vi "CallTransformation.vi"(8 "error in (no error)":errorcluster, 11 "TCP Network Connection in":refnum<k5>) -> (0 "error out":errorcluster, 2 "CallTrafoCluster":T1, 3 "TCP Network Connection out":refnum<k5>, 5 "Respond":string[](array[string]), 7 "Command":string)   [LabVIEW 2017]
uses:
  AT901 API/Structures/Struct CallTrafo.ctl
  AT901 API/TypeDefinitions/ES_DataType.ctl
  AT901 API/TypeDefinitions/ES_Command.ctl
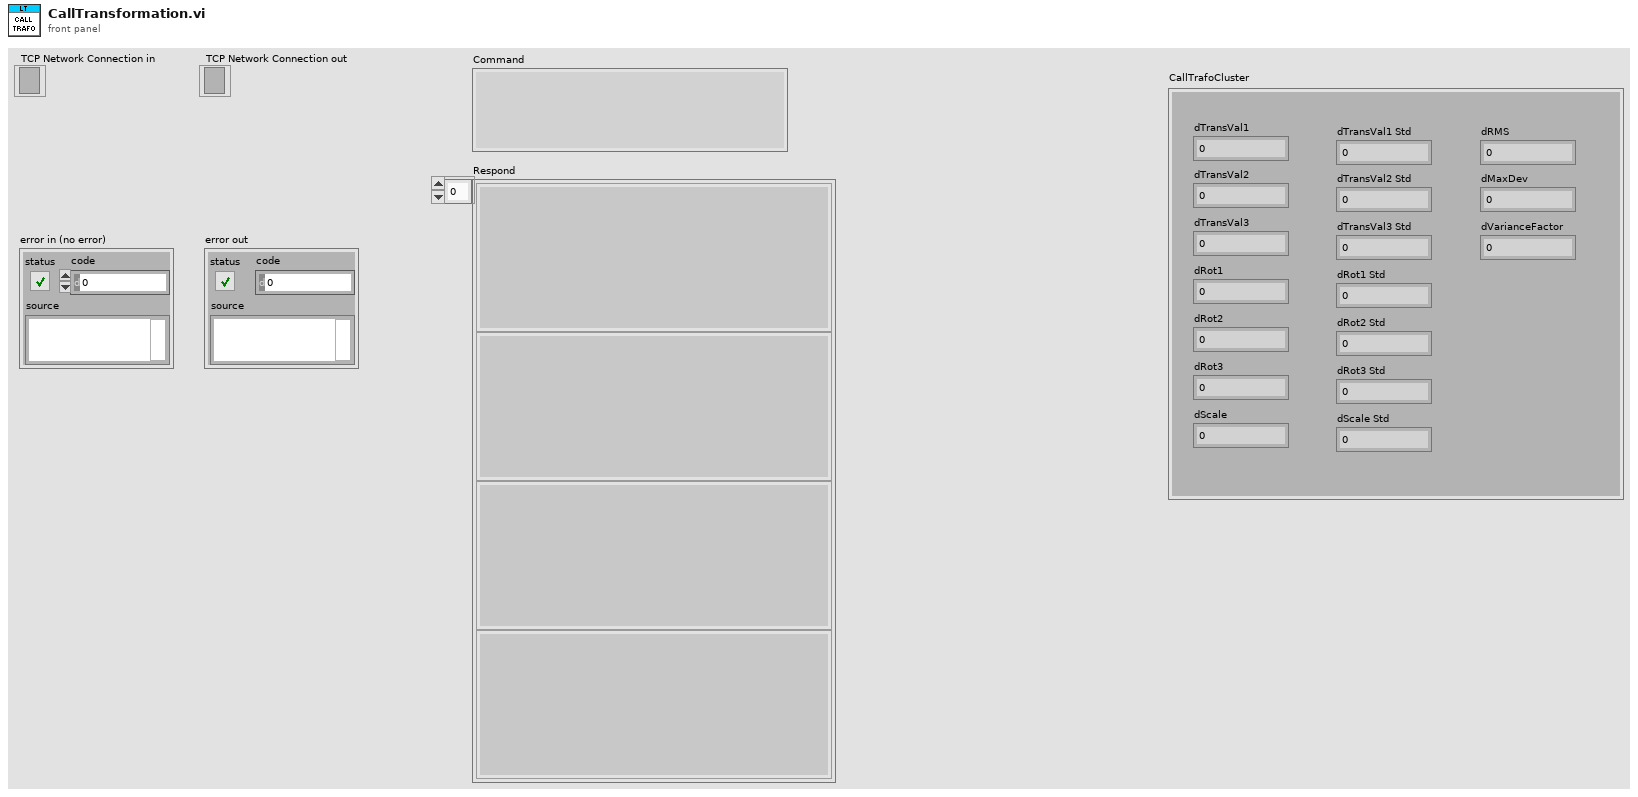
[diagram p1: front panel]
types:
  T1 = typedef "Struct CallTrafo.ctl" = cluster{"dTransVal1":dbl, "dTransVal2":dbl, "dTransVal3":dbl, "dRot1":dbl, "dRot2":dbl, "dRot3":dbl, "dScale":dbl, "dTransVal1 Std":dbl, "dTransVal2 Std":dbl, "dTransVal3 Std":dbl, "dRot1 Std":dbl, "dRot2 Std":dbl, "dRot3 Std":dbl, "dScale Std":dbl, "dRMS":dbl, "dMaxDev":dbl, "dVarianceFactor":dbl}
  T2 = typedef "ES_Command.ctl" = enum32{"ES_C_ExitApplication", "ES_C_GetSystemStatus", "ES_C_GetTrackerStatus", "ES_C_SetTemperatureRange", "ES_C_GetTemperatureRange", "ES_C_SetUnits", "ES_C_GetUnits", "ES_C_Intialize", "ES_C_ReleaseMotors", "ES_C_ActivateCameraView", "ES_C_Park", "ES_C_SwitchLaser", "ES_C_SetStationOriantationParams", "ES_C_GetStationOrientationParams", "ES_C_SetTransformationParams", "ES_C_GetTransformationParams", "ES_C_SetBoxRegionParams", "ES_C_GetBoxRegionParams", "ES_C_SetSphereRegionParams", "ES_C_GetSphereRegionParams", "ES_C_SetEnvironmentParams", "ES_C_GetEnvironmentParams", "ES_C_SetRefractionParams", "ES_C_GetRefractionParams", "ES_C_SetMeasurementMode", "ES_C_GetMeasurementMode", "ES_C_SetCoordinateSystemType", "ES_C_GetCoordinateSystemType", "ES_C_SetStationaryModeParams", "ES_C_GetStationaryModeParams", "ES_C_SetContinuousTimeModeParams", "ES_C_GetContinuousTimeModeParams", "ES_C_SetContinuousDistanceModeParams", "ES_C_GetContinuousDistanceModeParams", "ES_C_SetSphereCenterModeParams", "ES_C_GetSphereCenterModeParams", "ES_C_SetCircleCenterModeParams", "ES_C_GetCircleCenterModeParams", "ES_C_SetGridModeParams", "ES_C_GetGridModeParams", "ES_C_SetReflector", "ES_C_GetReflector", "ES_C_GetReflectors", "ES_C_SetSearchParams", "ES_C_GetSearchParams", "ES_C_SetAdmParams", "ES_C_GetAdmParams", "ES_C_SetSystemSettings", "ES_C_GetSystemSettings", "ES_C_StartMeasurement", "ES_C_Start6DMeasurement", "ES_C_StartNivelMeasurement", "ES_C_StopMeasurement", "ES_C_ChangeFace", "ES_C_GoBirdBath", "ES_C_GoPosition", "ES_C_GoPositionHVD", "ES_C_PositionRelativeHV", "ES_C_PointLaser", "ES_C_PointLaserHVD", "ES_C_MoveHV", "ES_C_GoNivelPosition", "ES_C_GoLastMeasuredPoint", "ES_C_FindReflector", "ES_C_Unknown", "ES_C_LookForTarget", "ES_C_GetDirection", "ES_C_CallOrientToGravity", "ES_C_ClearTransformationNominalPointList", "ES_C_ClearTransformationActualPointList", "ES_C_AddTransformationNominalPoint", "ES_C_AddTransformationActualPoint", "ES_C_SetTransformationInputParams", "ES_C_GetTransformationInputParams", "ES_C_CallTransformation", "ES_C_GetTransformedPoints", "ES_C_ClearDerivePointList", "ES_C_AddDrivePoint", "ES_C_CallIntermediateCompensation", "ES_C_SetCompensation", "ES_C_SetStatisticMode", "ES_C_GetStatisticMode", "ES_C_GetStillImage", "ES_C_SetCameraParams", "ES_C_GetCameraParams", "ES_C_GetCompensation", "ES_C_GetCompensations", "ES_C_CheckBirdBath", "ES_C_GetTrackerDiagnostics", "ES_C_GetADMInfo", "ES_C_GetTPInfo", "ES_C_GetNivelInfo", "ES_C_SetLaserOnTimer", "ES_C_GetLaserOnTimer", "ES_C_ConvertDisplayCoordinates", "ES_C_GorBirdBath2", "ES_C_SetTriggerSource", "ES_C_GetTriggerSource", "ES_C_GetFace", "ES_C_GetCameras", "ES_C_GetCamera", "ES_C_SetMeasurementCameraMode", "ES_C_GetMeasurementCameraMode", "ES_C_GetProbes", "ES_C_GetProbe", "ES_C_GetTipAdapters", "ES_C_GetTipAdapter", "ES_C_GetTCamToTrackerCompensations", "ES_C_GetTCamToTrackerCompensation", "ES_C_SetTCamToTrackerCompensation", "ES_C_GetProbeCompensations", "ES_C_GetProbeCompensation", "ES_C_SetProbeCompensation", "ES_C_GetTipToProbeCompensations", "ES_C_GetTipToProbeCompensation", "ES_C_SetExternTriggerParams", "ES_C_GetExternTriggerParams", "ES_C_GetErrorEllipsoid", "ES_C_GetMeasurementCameraInfo", "ES_C_GetMeasurementProbeInfo", "ES_C_SetLongSystemParameter", "ES_C_GetLongSystemParameter", "ES_C_GetMeasurementStatusInfo", "ES_C_GetCompensations2", "ES_C_GetCurrentPrismPosition", "ES_C_SetDoubleSystemParameter", "ES_C_GetDoubleSystemParameter", "ES_C_GetObjectTemperature", "ES_C_GetTriggerBoardInfo", "ES_C_GetOverviewCameraInfo", "ES_C_ClearCommandQueue", "ES_C_GetADMInfo2", "ES_C_GetTrackerInfo", "ES_C_GetNivelInfo2", "ES_C_RestoreStartupConditions", "ES_C_GoAndMeasure", "ES_C_GetTipToProbeCompensation2", "SetPowerLockMode", "GetPowerLockMode", "SetPowerLockFunctionAvailable", "GetPowerLockFunctionAvailable"}
  T3 = typedef "ES_DataType.ctl" = enum32{"ES_DT_Command", "ES_DT_Error", "ES_DT_SingleMeasResult", "ES_DT_MultiMeasResult", "ES_DT_StationaryProbeMeasResult", "ES_DT_ContinuousProbeMeasResult", "ES_DT_NivelResult", "ES_DT_ReflectorPosResult", "ES_DT_SystemStatusChange", "ES_DT_SingleMeasResult2", "ES_DT_MultiMeasResult2", "ES_DT_ProbePosResult"}
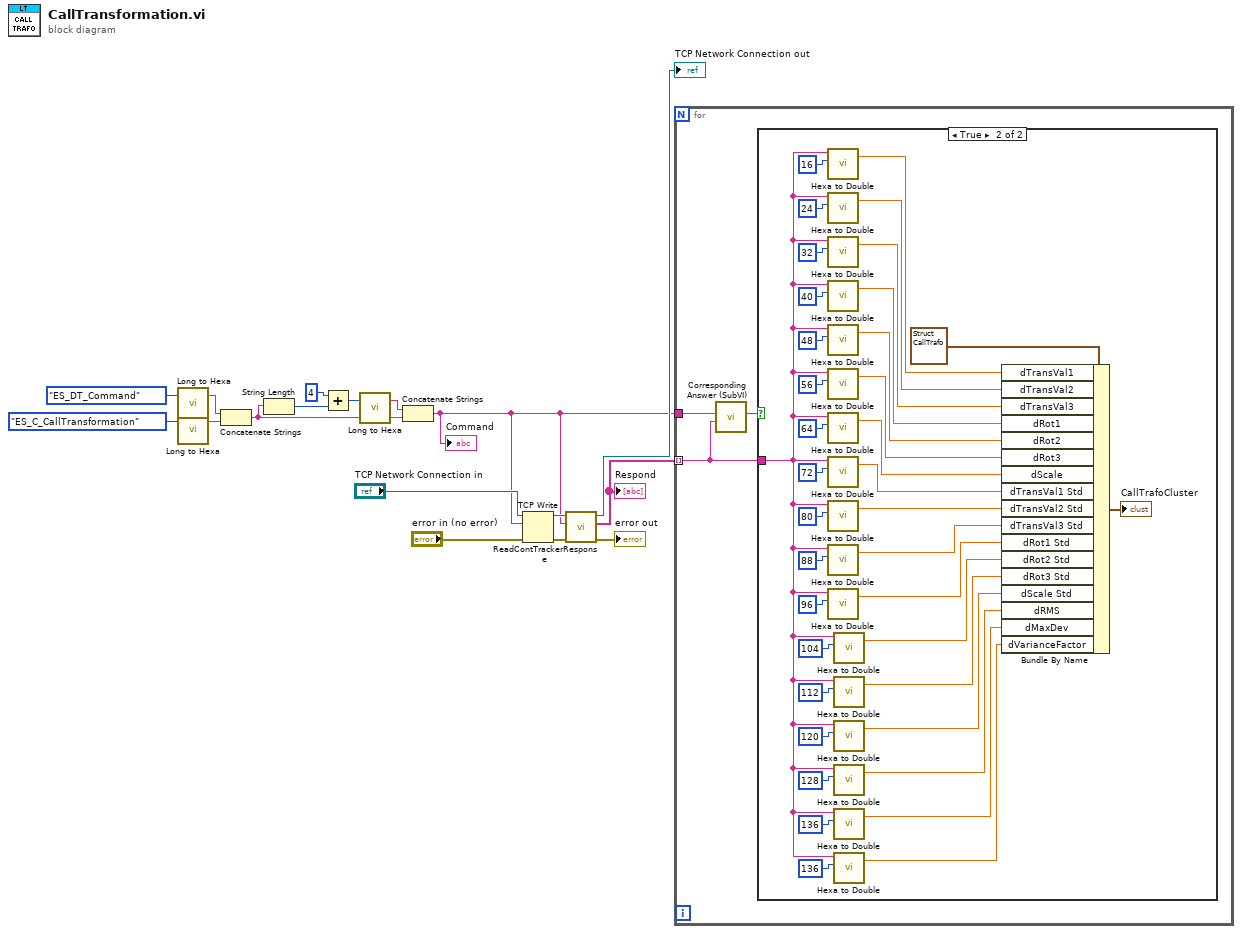
[diagram p0: block diagram]
diagram:
  n1 = call "Long to Hexa.vi"("Long"=ES_DataType."ES_DT_Command" ("ES_DataType")) -> ("Hexa"=w10:string)  [unwired: 2 in]
  n2 = call "Long to Hexa.vi"("Long"=ES_Command."ES_C_CallTransformation" ("ES_Command")) -> ("Hexa"=w11:string)  [unwired: 2 in]
  n3 = Concatenate Strings(w10, w11) -> (w8:string)
  n4 = String Length(string=w8) -> (length=w5:i32)
  n5 = Add(x=4 ("Index"), y=w5) -> (x+y=w7:i32)
  n6 = call "Long to Hexa.vi"("Long"=w7) -> ("Hexa"=w9:string)  [unwired: 2 in]
  n7 = Concatenate Strings(w9, w8) -> (w1:string)
  "Command" <- w1
  n8 = TCP Write(connection ID="TCP Network Connection in", data in=w1, error in (no error)="error in (no error)") -> (connection ID out=w12:refnum<k5>, error out=w14:errorcluster)  [unwired: 1 in, 1 out]
  n9 = call "ReadContTrackerResponse.vi"("error in (no error)"=w14, "Command"=w1, "TCP Network Connection in"=w12) -> ("error out"=→"error out":errorcluster, "Respond"=w2:string[], "TCP Network Connection out"=→"TCP Network Connection out":refnum<k5>)  [unwired: 6 in]
  "Respond" <- w2
  n10 = for {
    tunnel: w2 -> [w18] mode=indexing
    tunnel: w1 -> [w20]
    n11 = call "Corresponding Answer (SubVI).vi"("Command"=w20, "Tracker Response"=w18) -> ("Boolean"=w19:bool)  [unwired: 8 in]
    n12 = case shown="True" w19 {
      tunnel: w18 -> [_ w22]
      frame False {
      }
      frame True {
        n13 = call "Hexa to Double.vi"("Hexa"=w22, "Index"=16) -> ("Double"=w40:dbl)  [unwired: 4 in]
        n14 = call "Hexa to Double.vi"("Hexa"=w22, "Index"=24) -> ("Double"=w39:dbl)  [unwired: 4 in]
        n15 = call "Hexa to Double.vi"("Hexa"=w22, "Index"=32) -> ("Double"=w38:dbl)  [unwired: 4 in]
        n16 = call "Hexa to Double.vi"("Hexa"=w22, "Index"=40) -> ("Double"=w37:dbl)  [unwired: 4 in]
        n17 = call "Hexa to Double.vi"("Hexa"=w22, "Index"=48) -> ("Double"=w36:dbl)  [unwired: 4 in]
        n18 = call "Hexa to Double.vi"("Hexa"=w22, "Index"=56) -> ("Double"=w35:dbl)  [unwired: 4 in]
        n19 = call "Hexa to Double.vi"("Hexa"=w22, "Index"=64) -> ("Double"=w34:dbl)  [unwired: 4 in]
        n20 = call "Hexa to Double.vi"("Hexa"=w22, "Index"=72) -> ("Double"=w33:dbl)  [unwired: 4 in]
        n21 = call "Hexa to Double.vi"("Hexa"=w22, "Index"=80) -> ("Double"=w32:dbl)  [unwired: 4 in]
        n22 = call "Hexa to Double.vi"("Hexa"=w22, "Index"=88) -> ("Double"=w31:dbl)  [unwired: 4 in]
        n23 = call "Hexa to Double.vi"("Hexa"=w22, "Index"=96) -> ("Double"=w30:dbl)  [unwired: 4 in]
        n24 = call "Hexa to Double.vi"("Hexa"=w22, "Index"=104) -> ("Double"=w29:dbl)  [unwired: 4 in]
        n25 = call "Hexa to Double.vi"("Hexa"=w22, "Index"=112) -> ("Double"=w28:dbl)  [unwired: 4 in]
        n26 = call "Hexa to Double.vi"("Hexa"=w22, "Index"=120) -> ("Double"=w27:dbl)  [unwired: 4 in]
        n27 = call "Hexa to Double.vi"("Hexa"=w22, "Index"=128) -> ("Double"=w26:dbl)  [unwired: 4 in]
        n28 = call "Hexa to Double.vi"("Hexa"=w22, "Index"=136) -> ("Double"=w25:dbl)  [unwired: 4 in]
        n29 = call "Hexa to Double.vi"("Hexa"=w22, "Index"=136) -> ("Double"=w23:dbl)  [unwired: 4 in]
        n30 = Bundle By Name(cluster=T1 {"dTransVal1"=0.0, "dTransVal2"=0.0, "dTransVal3"=0.0, "dRot1"=0.0, "dRot2"=0.0, "dRot3"=0.0, "dScale"=0.0, "dTransVal1 Std"=0.0, "dTransVal2 Std"=0.0, "dTransVal3 Std"=0.0, "dRot1 Std"=0.0, "dRot2 Std"=0.0, "dRot3 Std"=0.0, "dScale Std"=0.0, "dRMS"=0.0, "dMaxDev"=0.0, "dVarianceFactor"=0.0} ("CallTrafoCluster"), "dTransVal1"=w40, "dTransVal2"=w39, "dTransVal3"=w38, "dRot1"=w37, "dRot2"=w36, "dRot3"=w35, "dScale"=w34, "dTransVal1 Std"=w33, "dTransVal2 Std"=w32, "dTransVal3 Std"=w31, "dRot1 Std"=w30, "dRot2 Std"=w29, "dRot3 Std"=w28, "dScale Std"=w27, "dRMS"=w26, "dMaxDev"=w25, "dVarianceFactor"=w23) -> (→"CallTrafoCluster":T1)
      }
    }
  }
